vi "Pack Message.vi"(8 "error in (no error)":errorcluster, 11 "Car Wash Option Started in":refnum<class "Car Wash Option Started.lvclass">) -> (0 "error out":errorcluster, 1 "Packed Message":string, 2 "Message Name":string, 3 "Car Wash Option Started out":refnum<class "Car Wash Option Started.lvclass">)   [LabVIEW 2016, in "CLD Exam - Car Wash.lvlib" / "Car Wash Option Started.lvclass"]
uses:
  Car Wash Option Started.lvclass
  Mediator/Classes/Message Data Interface/Data Message Interface.lvclass
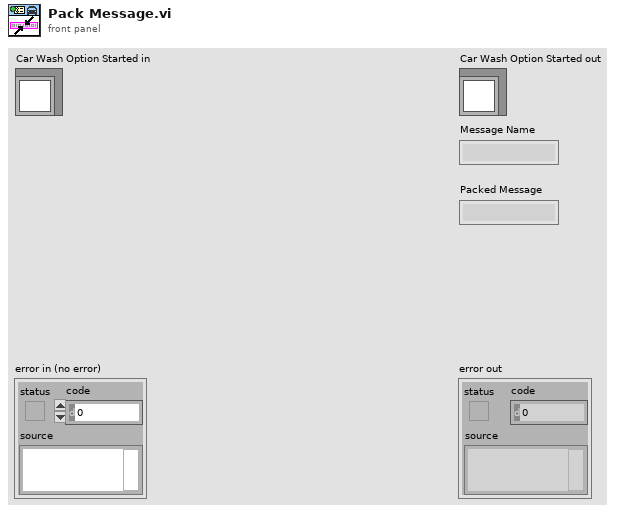
[diagram p1: front panel]
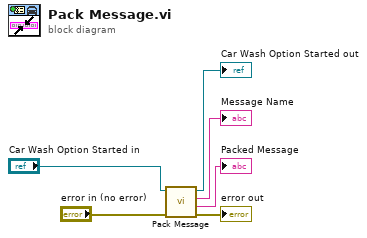
[diagram p0: block diagram]
diagram:
  n1 = call-parent "Pack Message.vi"("error in (no error)"="error in (no error)", "Data Message Interface in"="Car Wash Option Started in") -> ("error out"=→"error out":errorcluster, "Packed Message"=→"Packed Message":string, "Message Name"=→"Message Name":string, "Data Message Interface out"=→"Car Wash Option Started out":refnum<class "Car Wash Option Started.lvclass">)  [unwired: 6 in]
